vi "Wait.vi"(8 "error in":errorcluster, 11 "Purge Time (s)":u32) -> (0 "error out":errorcluster)   [LabVIEW 2017, in "Controller.lvlib"]
uses:
  Controller.lvlib
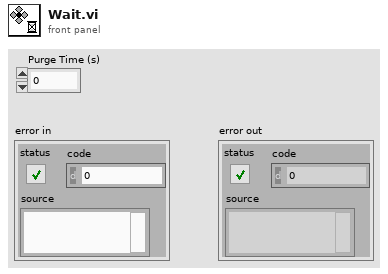
[diagram p1: front panel]
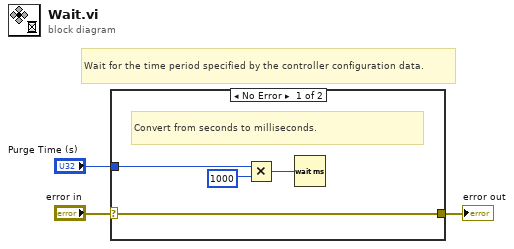
[diagram p0: block diagram]
diagram:
  # "Wait for the time period specified by the controller configuration data."
  n1 = case shown="No Error" "error in" {
    selector: "error in" -> [w4 w8]
    tunnel: "Purge Time (s)" -> [w5 _]
    tunnel: [w4 w8] -> w1
    frame No Error {
      # "Convert from seconds to milliseconds."
      n2 = Multiply(x=w5, y=u32 1000 ("x")) -> (x*y=w6:u32)
      n3 = Wait (ms)(milliseconds to wait=w6) -> ()  [unwired: 1 out]
    }
    frame Error {
    }
  }
  "error out" <- w1
